vi "PCsensor.GetTandH.vi"(8 "error in (no error)":errorcluster, 11 "PCsensor Device Handle":i64) -> (0 "error out":errorcluster, 2 "Humidity":dbl, 3 "Temperature":dbl)   [LabVIEW 2019, in "TEMPerHUM.lvlib"]
uses:
  TEMPerHUM.lvlib
  SMOs/TEMPerHUM/RDingUSB.dll
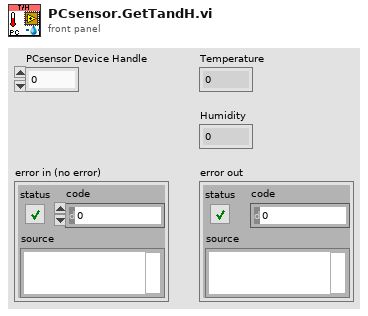
[diagram p1: front panel]
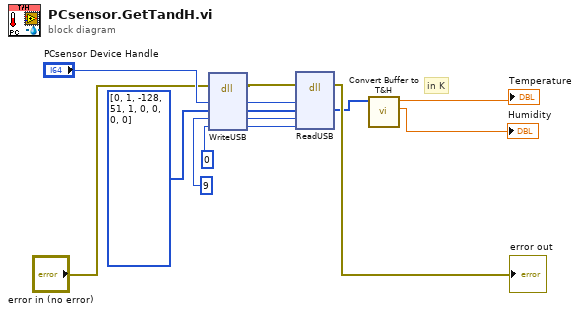
[diagram p0: block diagram]
diagram:
  # "in K"
  n1 = dll-call lib="C:/Users/Ranjani/Documents/GitHub/Temperhum-Instrument/lvsrc/SMOs/TEMPerHUM/RDingUSB.dll" fn="WriteUSB"(error in="error in (no error)", "deviceHandle"="PCsensor Device Handle", "buffer"=i8[] [0, 1, -128, 51, 1, 0, 0, 0, 0] ("Array"), "bytesCount"=9, "number0fBytesWrite"=u64 0) -> (error out=w6:errorcluster, "deviceHandle"=w4:i64, "buffer"=w3:i8[], "bytesCount"=w2:i32, "number0fBytesWrite"=w1:u64)  [unwired: 3 in, 1 out]
  n2 = dll-call lib="C:/Users/Ranjani/Documents/GitHub/Temperhum-Instrument/lvsrc/SMOs/TEMPerHUM/RDingUSB.dll" fn="ReadUSB"(error in=w6, "deviceHandle"=w4, "buffer"=w3, "bytesCount"=w2, "number0fBytesRead"=w1) -> (error out=→"error out":errorcluster, "buffer"=w11:u8[])  [unwired: 6 in, 1 out]
  n3 = call "Convert Buffer to T&H.vi"("buffer"=w11) -> ("Humidity"=→"Humidity":dbl, "Temperature"=→"Temperature":dbl)  [unwired: 9 in]
